vi "Cmd Get Datetime Parameter Value (C).vi"(6 "error in (no error)":errorcluster, 7 "type":string, 8 "parameter index":variant, 9 "command reference":T1) -> (0 "error out":errorcluster, 1 "value":string, 3 "command reference out":T1)   [LabVIEW 2020, in "NI_Database_API.lvlib"]
doc: "Retrieves the value of the parameter specified by the <B>parameter index</B> input in the command or command-recordset. The <B>parameter index</B> can be either the zero-indexed position of the parameter in the command or the name of the parameter. Wire data to the <B>type</B> input to determine the polymorphic instance to use or manually select the instance."
uses:
  <vilib>/addons/database/NI_Database_API.lvlib
  <vilib>/addons/database/Command.llb/Cmd ObjectReference.ctl
  <vilib>/addons/database/_DB Variant To Data/Database Variant To Data.xnode
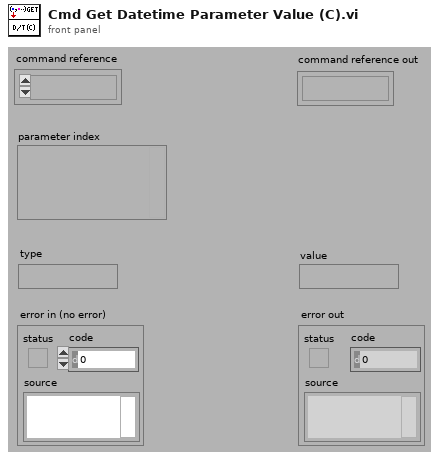
[diagram p1: front panel]
types:
  T1 = typedef "NI_Database_API.lvlib/Cmd ObjectReference.ctl" = refnum<k1>
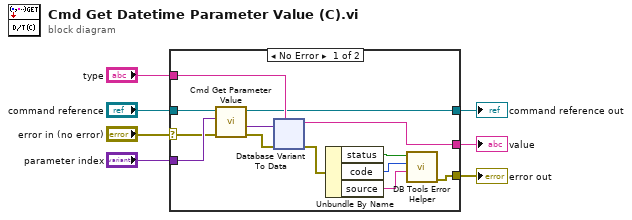
[diagram p0: block diagram]
diagram:
  n1 = case shown="No Error" "error in (no error)" {
    selector: "error in (no error)" -> [w8 w54]
    tunnel: "type" -> [w20 _]
    tunnel: [w19 _] -> w6
    tunnel: "parameter index" -> [w18 _]
    tunnel: "command reference" -> [w17 w53]
    tunnel: [w15 w53] -> w3
    tunnel: [w10 w54] -> w2
    frame No Error {
      n2 = call <vilib>:"Cmd Get Parameter Value.vi"("error in (no error)"=w8, "parameter index"=w18, "command reference"=w17) -> ("error out"=w16:errorcluster, "value"=w9:variant, "command reference out"=w15:T1)  [unwired: 2 out]
      n3 = xnode "Database Variant To Data"("database variant"=w9, "error in"=w16, "type"=w20) -> ("data"=w19:string, "error out"=w11:errorcluster)
      n4 = Unbundle By Name(w11) -> ("status"=w13:bool, "code"=w12:i32, "source"=w14:string)
      n5 = call <vilib>:"DB Tools Error Helper.vi"("source"=w14, "code"=w12, "status"=w13) -> ("error out"=w10:errorcluster)  [unwired: 1 in, 7 out]
    }
    frame Error {
    }
  }
  "error out" <- w2
  "command reference out" <- w3
  "value" <- w6
